vi "Generator_Dataset_Raw.vi"() -> ()   [LabVIEW 2025]
uses:
  <vilib>/Utility/file.llb/Write Delimited Spreadsheet (DBL).vi
panel:
  in  "Path":path
  in  "Numar pacienti":dbl
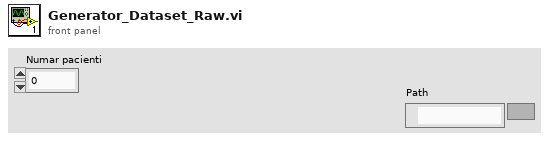
[diagram p1: front panel]
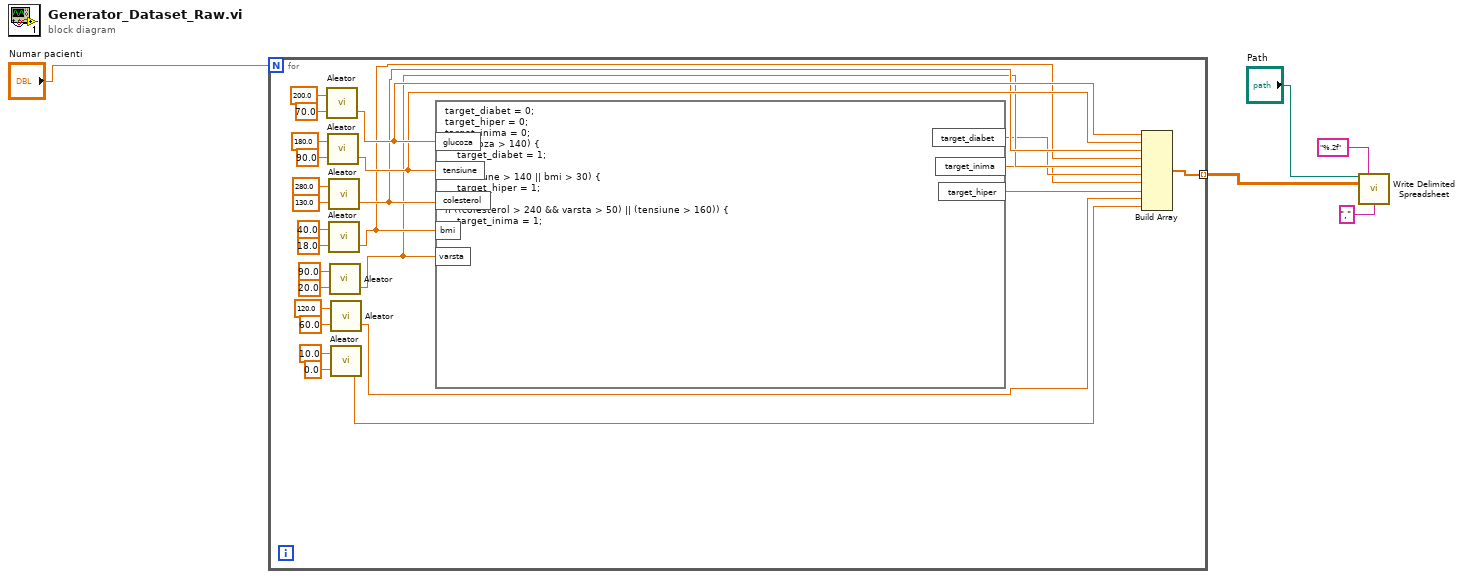
[diagram p0: block diagram]
diagram:
  n1 = for {
    N: "Numar pacienti" -> [_]
    tunnel: [w12] -> w4 mode=indexing
    n2 = call "Aleator.vi"("minim"=70.0, "maxim"=200.0) -> ("valoare generata"=w30:dbl)  [unwired: 1 in]
    n3 = call "Aleator.vi"("minim"=90.0, "maxim"=180.0) -> ("valoare generata"=w29:dbl)  [unwired: 1 in]
    n4 = call "Aleator.vi"("minim"=130.0, "maxim"=280.0) -> ("valoare generata"=w28:dbl)  [unwired: 1 in]
    n5 = call "Aleator.vi"("minim"=18.0, "maxim"=40.0) -> ("valoare generata"=w27:dbl)  [unwired: 1 in]
    n6 = call "Aleator.vi"("minim"=20.0, "maxim"=90.0) -> ("valoare generata"=w26:dbl)  [unwired: 1 in]
    n7 = call "Aleator.vi"("minim"=60.0, "maxim"=120.0) -> ("valoare generata"=w7:dbl)  [unwired: 1 in]
    n8 = call "Aleator.vi"("minim"=0.0, "maxim"=10.0) -> ("valoare generata"=w6:dbl)  [unwired: 1 in]
    n9 = formula code="target_diabet = 0;\ntarget_hiper = 0;\ntarget_inima = 0;\nif (glucoza > 140) {\n    target_diabet = 1;\n}\nif (tensiune > 140 || bmi > 30) {\n    target_hiper = 1;\n}\nif ((colesterol > 240 && varsta > 50) || (tensiune > 160)) {\n    target_inima = 1;\n}"("glucoza"=w30, "tensiune"=w29, "colesterol"=w28, "bmi"=w27, "varsta"=w26) -> ("target_diabet"=w25:dbl, "target_inima"=w24:dbl, "target_hiper"=w23:dbl)
    n10 = Build Array(w30, w29, w28, w27, w26, w25, w24, w23, w7, w6) -> (w12:dbl[])
  }
  n11 = call-poly <vilib>:"Write Delimited Spreadsheet.vi"("file path (dialog if empty)"="Path", "format (%.3f)"="%.2f", "2D data"=w4, "delimiter (\\t)"="," ("delimiter (\\t)")) -> ()  [unwired: 10 in, 2 out]
